vi "Data Sensor.vi"(0 "VISA resource name":refnum<visa-resource-name>, 7 "Input (0: A)":u16(ring) items=["A", "B", "C", "D"], 11 "error in (no error)":errorcluster) -> (4 "VISA resource name out":refnum<visa-resource-name>, 6 "Celsius Reading":dbl min=-273.16 max=1372.0 step=1e-05 format="%^.5e", 8 "Kelvin Reading":dbl min=0.0 max=1645.0 step=1e-05 format="%^.5e", 10 "Sensor Units Reading":dbl min=-7.5 max=300000.0 step=1e-05 format="%^.5e", 15 "error out":errorcluster)   [LabVIEW 2019, in "Lake Shore Cryotronics 340.lvlib"]
doc: "This VI querys the instrument for an inputs sensor reading in Celsius, Kelvin, and Sensor Units."
uses:
  Lake Shore Cryotronics 340.lvlib
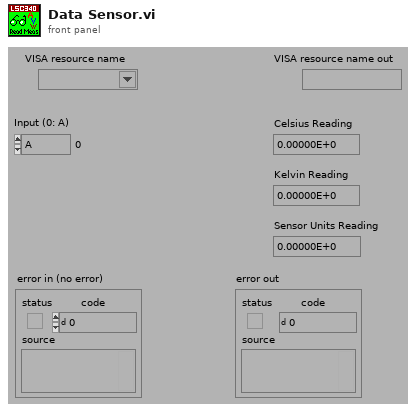
[diagram p1: front panel]
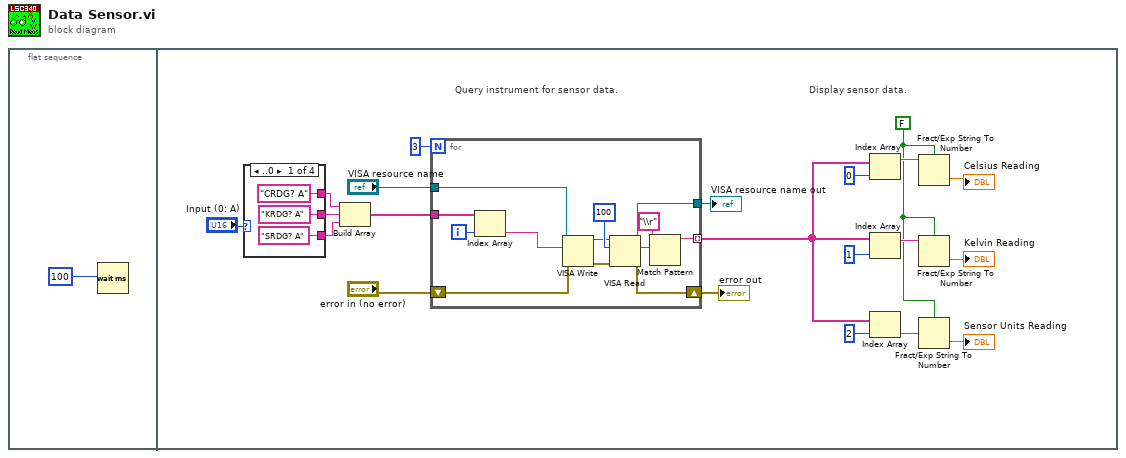
[diagram p0: block diagram]
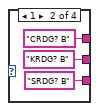
[diagram p2: hidden frame]
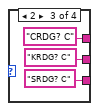
[diagram p3: hidden frame]
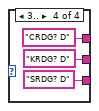
[diagram p4: hidden frame]
diagram:
  n1 = flat-sequence {
    frame #0 {
      n2 = Wait (ms)(milliseconds to wait=100) -> ()  [unwired: 1 out]
    }
    frame #1 {
      w2 = FALSE ("use system decimal point (T)")
      # "Query instrument for sensor data."
      # "Display sensor data."
      n3 = case shown="..0" "Input (0: A)" {
        tunnel: ["CRDG? A" "CRDG? B" "CRDG? C" "CRDG? D"] -> w11
        tunnel: ["KRDG? A" "KRDG? B" "KRDG? C" "KRDG? D"] -> w10
        tunnel: ["SRDG? A" "SRDG? B" "SRDG? C" "SRDG? D"] -> w9
        frame ..0 {
        }
        frame 1 {
        }
        frame 2 {
        }
        frame 3.. {
        }
      }
      n4 = Build Array(w11, w10, w9) -> (w12:string[])
      n5 = for {
        N: 3 -> [_]
        tunnel: w12 -> [w44]
        shift-right: [w41] -> w5
        shift-left: "error in (no error)" -> [w42]
        tunnel: [w40] -> w4
        tunnel: "VISA resource name" -> [w39]
        tunnel: [w37] -> w3 mode=indexing
        i -> [w43]
        n6 = Index Array(array=w44, index=w43) -> (element=w35:string)
        n7 = VISA Write(VISA resource name=w39, write buffer=w35, error in (no error)=w42) -> (VISA resource name out=w36:refnum<visa-resource-name>, error out=w47:errorcluster)  [unwired: 1 out]
        n8 = VISA Read(VISA resource name=w36, byte count=100, error in (no error)=w47) -> (VISA resource name out=w40:refnum<visa-resource-name>, read buffer=w45:string, error out=w41:errorcluster)  [unwired: 1 out]
        n9 = Match Pattern(string=w45, regular expression="\\r") -> (before substring=w37:string)  [unwired: 1 in, 3 out]
      }
      "VISA resource name out" <- w4
      "error out" <- w5
      n10 = Index Array(array=w3, index=0) -> (element=w17:string)
      n11 = Index Array(array=w3, index=1) -> (element=w18:string)
      n12 = Index Array(array=w3, index=2) -> (element=w19:string)
      n13 = Fract/Exp String To Number(use system decimal point (T)=w2, string=w17) -> (number=→"Celsius Reading":dbl)  [unwired: 2 in, 1 out]
      n14 = Fract/Exp String To Number(use system decimal point (T)=w2, string=w18) -> (number=→"Kelvin Reading":dbl)  [unwired: 2 in, 1 out]
      n15 = Fract/Exp String To Number(use system decimal point (T)=w2, string=w19) -> (number=→"Sensor Units Reading":dbl)  [unwired: 2 in, 1 out]
    }
  }
